vi "Relative Path Tag--constant.vi"() -> (3 "Relative Path Tag":string)   [LabVIEW 2021]
doc: "CONSTANT VI - defines the user VI tag for the relative path status\n\n<b>Code Developed By:</b>\nDaniel Coons\nTechnology Service Corporation\nwww.tsc.com/atcs"
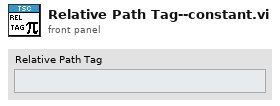
[diagram p1: front panel]
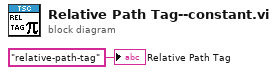
[diagram p0: block diagram]
diagram:
  "Relative Path Tag" <- "relative-path-tag" ("Theme Path Tag")
